vi "Measurement Logic.vi"() -> ()   [LabVIEW 2021, in "AC Dual Channel_Audio ADC.lvlib"]
uses:
  AC Dual Channel_Audio ADC.lvlib
  Measurement Configuration.ctl
  Measurement Results.ctl
  <vilib>/MeasurementLink/MeasurementLink Measurement Server/Measure Call Context/Measure Call Context.lvclass
  shared/controls/Sync Commands.ctl
  <vilib>/DAQmx/create/channels.llb/DAQmx Create Channel (AO-FuncGen).vi
  <vilib>/PDM Acquisition Toolkit/host/API/Public/Start/Start PCM Input Task.vi
  <vilib>/PDM Acquisition Toolkit/host/API/Public/Read/Read PCM Input Waveform.vi
  <vilib>/PDM Acquisition Toolkit/host/API/Public/Clear/Clear PCM Input Task.vi
  shared/controls/Audio ADC Controls.lvlib
  shared/Audio ADC Shared.lvlib
  <vilib>/PDM Acquisition Toolkit/host/API/PDM Acquisition Toolkit.lvlib
panel:
  out "measure call context out":refnum<class "Measure Call Context.lvclass">
  in  "measure call context in":refnum<class "Measure Call Context.lvclass">
  out "measurement results":T1
  in  "measurement configuration":T2={"Band start"=20.0, "Band stop"=20000.0, "Weighting Filter"=enum."Linear", "Full scale range"=2.825, "Left channel name"="", "Right channel name"="", "Left channel analog source resource name"="", "Right channel analog source resource name"="", "Frequency"=1000.0, "Amplitude"=-1.0, "Protocol capture resource name"="", "Data line"=0, "Left acquisition channel"=0, "Right acquisition channel"=0, "Sample rate"=44100.0, "Measurement Duration"=0.1, "Frame sync edge for Channel 0"=enum."Falling", "Channel count per frame"=2, "Channel length"=32, "Bit depth"=24, "Channel 0 offset"=1, "Endianness"=enum."MSB First", "Data Justification"=enum."Left Justified", "Frame length"=64, "Frame sync pulse width"=32, "Bit clock edge  sync"=enum."Falling"} {"Frame length" format="%#_6ps"}
  out "error out":errorcluster
  in  "error in":errorcluster
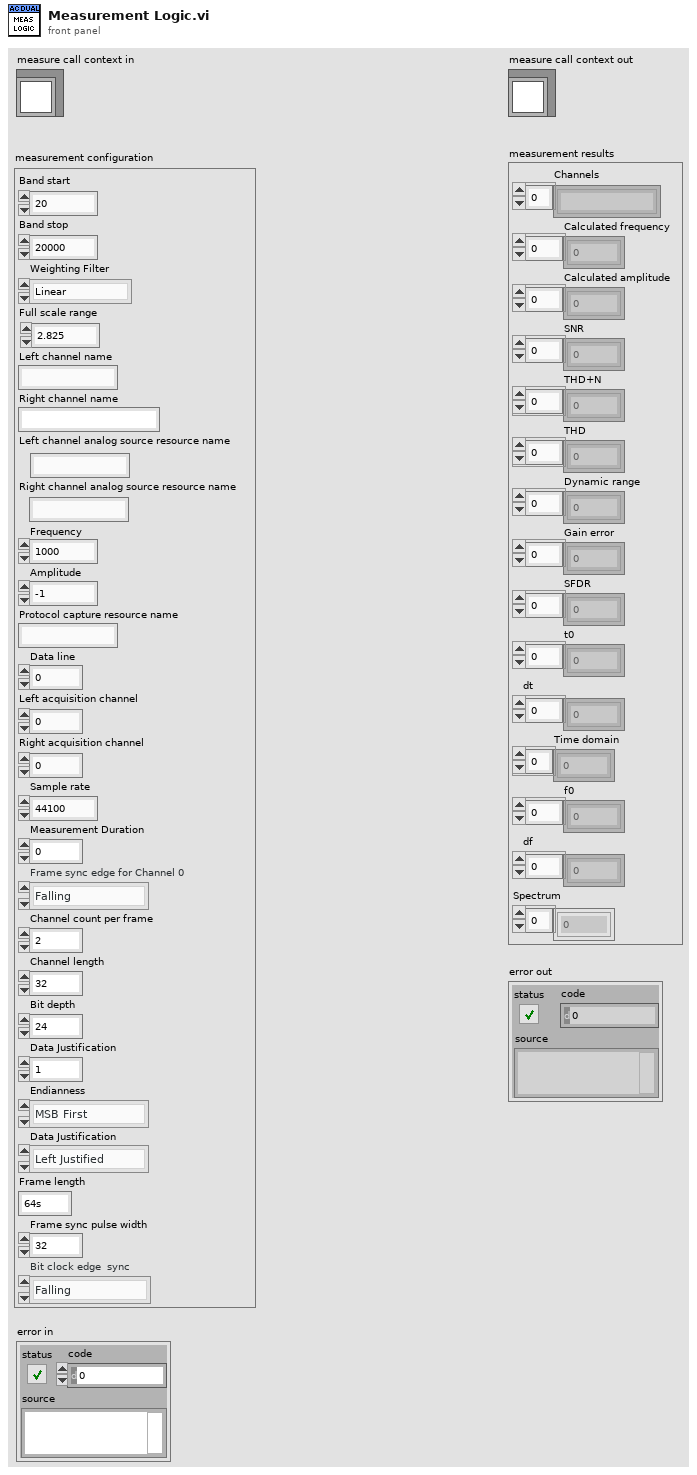
[diagram p1: front panel]
types:
  T1 = typedef "AC Dual Channel_Audio ADC.lvlib/Measurement Results.ctl" = cluster{"Channels":string[], "Calculated frequency":dbl[], "Calculated amplitude":dbl[], "SNR":dbl[], "THD+N":dbl[], "THD":dbl[], "Dynamic range":dbl[], "Gain error":dbl[], "SFDR":dbl[], "t0":dbl[], "dt":dbl[], "Time domain":dbl[], "f0":dbl[], "df":dbl[], "Spectrum":dbl[]}
  T2 = typedef "AC Dual Channel_Audio ADC.lvlib/Measurement Configuration.ctl" = cluster{"Band start":dbl, "Band stop":dbl, "Weighting Filter":enum32{"Linear", "A-weighting", "B-weighting", "C-weighting"}, "Full scale range":dbl, "Left channel name":string, "Right channel name":string, "Left channel analog source resource name":string, "Right channel analog source resource name":string, "Frequency":dbl, "Amplitude":dbl, "Protocol capture resource name":string, "Data line":i32, "Left acquisition channel":i32, "Right acquisition channel":i32, "Sample rate":dbl, "Measurement Duration":dbl, "Frame sync edge for Channel 0":enum32{"Rising", "Falling"}, "Channel count per frame":u32, "Channel length":u32, "Bit depth":u32, "Channel 0 offset":u32, "Endianness":enum32{"MSB First", "LSB First"}, "Data Justification":enum32{"Left Justified", "Right Justified"}, "Frame length":u32, "Frame sync pulse width":u32, "Bit clock edge  sync":enum32{"Rising", "Falling"}}
  T3 = typedef "audio adc controls.lvlib/Sync Commands.ctl" = enum16{"NoAction", "GenerationStarted", "AcquisitionCompleted", "GenerationErrored"}
  T4 = typedef "Audio ADC Controls.lvlib/Protocol Settings Dual Channel.ctl" = cluster{"Protocol capture resource name":string, "Data line":u16, "Channel":string, "Clock rate":u32, "Number of words":i32, "Sensitivity":dbl, "Frame sync edge for channel 0":enum32{"Rising", "Falling"}, "Channel count per frame":u8, "Channel length":u16, "Bit depth":u8, "Channel 0 offset":u16, "Endianness":enum32{"MSB First", "LSB First"}, "Data justification":enum32{"Left Justified", "Right Justified"}, "Frame length":u16, "Frame sync pulse width":u16, "Bit clock edge sync":enum32{"Rising", "Falling"}}
  T5 = typedef "PDM Acquisition Class Library.lvlib/PCM Input Task.lvclass/DVR PCM Input Task.ctl" = refnum<data-value>
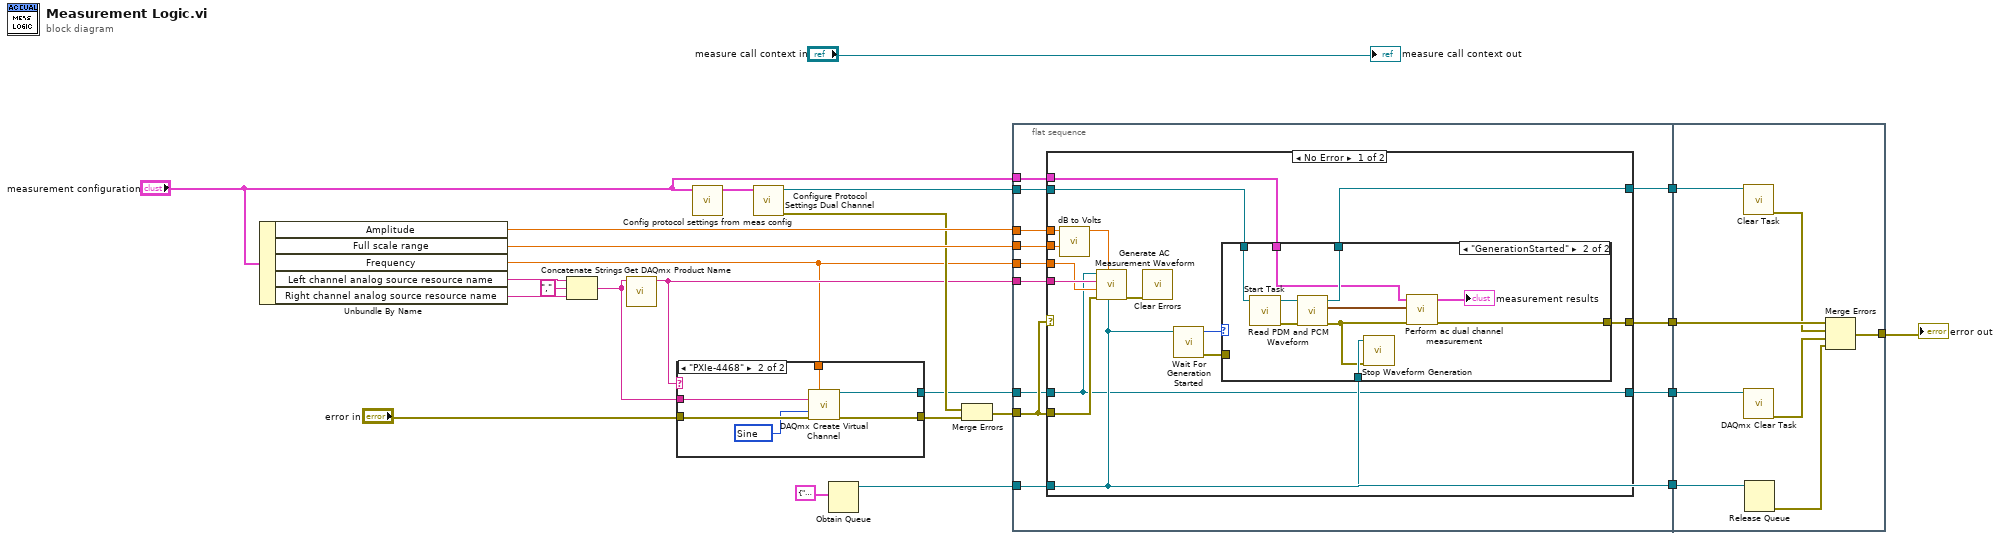
[diagram p0: block diagram]
diagram:
  n1 = Unbundle By Name("measurement configuration") -> ("Amplitude"=w19:dbl, "Full scale range"=w18:dbl, "Frequency"=w11:dbl, "Left channel analog source resource name"=w6:string, "Right channel analog source resource name"=w4:string)
  n2 = Concatenate Strings(w6, "," ("string"), w4) -> (w5:string)
  n3 = call "Get DAQmx Product Name.vi"("DAQmx resource name"=w5) -> ("DAQmx product type"=w12:string)  [unwired: 10 in]
  n4 = case shown="\"PXIe-4468\"" w12 {
    tunnel: w5 -> [_ w30]
    tunnel: "error in" -> [w25 w31]
    tunnel: [w25 w27] -> w16
    tunnel: w11 -> [_ w28]
    tunnel: [_ w26] -> w1
    frame Default {
    }
    frame "PXIe-4468" {
      w29 = 14751 items=["Sine"=14751, "Triangle"=14752, "Square"=14753, "Sawtooth"=14754] ("type")
      n5 = call-poly <vilib>:"DAQmx Create Virtual Channel.vi"("frequency"=w28, "physical channels"=w30, "type"=w29, "error in"=w31) -> ("task out"=w26:refnum<k21>, "error out"=w27:errorcluster)  [unwired: 10 in]
    }
  }
  n6 = call "Config protocol settings from meas config.vi"("measurement configuration"="measurement configuration") -> ("Protocol settings"=w8:T4)  [unwired: 10 in]
  n7 = call "Configure Protocol Settings Dual Channel.vi"("Protocol settings"=w8) -> ("error out"=w15:errorcluster, "PCM input task out"=w17:T5)  [unwired: 9 in]
  n8 = Obtain Queue(element data type=cluster{"Status":T3, "Error":errorcluster} {"Status"=enum."NoAction", "Error"={"status"=FALSE, "code"=0, "source"=""}}) -> (queue out=w13:refnum<queue>)  [unwired: 4 in, 2 out]
  n9 = Merge Errors(w15, w16) -> (w14:errorcluster)
  n10 = flat-sequence {
    tunnel: w19 -> [w43]
    tunnel: w18 -> [w42]
    tunnel: w13 -> [w40]
    tunnel: w14 -> [w34]
    tunnel: w17 -> [w41]
    tunnel: [w40] -> w23
    tunnel: [w38] -> w22
    tunnel: [w39] -> w21
    tunnel: w12 -> [w37]
    tunnel: w11 -> [w36]
    tunnel: "measurement configuration" -> [w35]
    tunnel: [w33] -> w2
    tunnel: w1 -> [w32]
    tunnel: w23 -> [w81]
    tunnel: w22 -> [w80]
    tunnel: w21 -> [w79]
    tunnel: [w75] -> w9
    tunnel: w2 -> [w74]
    frame #0 {
      n11 = case shown="No Error" w34 {
        selector: w34 -> [_ w72]
        tunnel: w43 -> [w58 _]
        tunnel: w42 -> [w57 _]
        tunnel: w34 -> [w54 _]
        tunnel: w41 -> [w53 w73]
        tunnel: w40 -> [w50 _]
        tunnel: [w49 w72] -> w39
        tunnel: [w48 w73] -> w38
        tunnel: w37 -> [w47 _]
        tunnel: w36 -> [w46 _]
        tunnel: w35 -> [w45 _]
        tunnel: [w44 w71] -> w33
        tunnel: w32 -> [w44 w71]
        frame No Error {
          n12 = call "dB to Volts.vi"("Full scale range"=w57, "Voltage(dB)"=w58) -> ("Voltage(volts)"=w56:dbl)  [unwired: 9 in]
          n13 = call "Generate AC Measurement Waveform.vi"("hardware commands sync queue"=w50, "Voltage(volts)"=w56, "error in"=w54, "Frequency"=w46, "DAQmx product name"=w47, "DSG task in"=w44) -> ("error out"=w55:errorcluster)  [unwired: 4 in, 1 out]
          n14 = call <vilib>:"Clear Errors.vi"("error in (no error)"=w55) -> ()  [unwired: 5 in, 2 out]
          n15 = call "Wait For Generation Started.vi"("hardware commands sync queue"=w50) -> ("error out"=w51:errorcluster, "Status"=w52:T3)  [unwired: 9 in]
          n16 = case shown="\"GenerationStarted\"" w52 {
            tunnel: w53 -> [w59 w68]
            tunnel: [w60 w65] -> w49
            tunnel: w51 -> [w60 _]
            tunnel: [w59 w67] -> w48
            tunnel: w50 -> [_ w66]
            tunnel: w45 -> [_ w63]
            frame Default {
            }
            frame "GenerationStarted" {
              n17 = call-poly <vilib>:"Start Task.vi"("PCM input task in"=w68) -> ("error out"=w70:errorcluster, "PCM input task out"=w69:T5)  [unwired: 9 in]
              n18 = call-poly <vilib>:"Read PDM and PCM Waveform.vi"("error in"=w70, "PCM input task In"=w69) -> ("error out"=w62:errorcluster, "PCM waveforms"=w64:waveform(dbl)[], "PCM input task out"=w67:T5)  [unwired: 4 in, 3 out]
              n19 = call "Stop Waveform Generation.vi"("error in (no error)"=w62, "Hw sync command Q"=w66) -> ()  [unwired: 10 in]
              n20 = call "Perform ac dual channel measurement.vi"("error in"=w62, "I2S waveforms"=w64, "measurement configuration"=w63) -> ("error out"=w65:errorcluster, "measurement results"=→"measurement results":T1)  [unwired: 7 in]
            }
          }
        }
        frame Error {
        }
      }
    }
    frame #1 {
      n21 = call-poly <vilib>:"Clear Task.vi"("PCM input task in"=w80) -> ("error out"=w78:errorcluster)  [unwired: 10 in]
      n22 = call <vilib>:"DAQmx Clear Task.vi"("task in"=w74) -> ("error out"=w77:errorcluster)  [unwired: 14 in]
      n23 = Release Queue(queue=w81) -> (error out=w76:errorcluster)  [unwired: 2 in, 2 out]
      n24 = Merge Errors(w79, w78, w77, w76) -> (w75:errorcluster)
    }
  }
  "error out" <- w9
  "measure call context out" <- "measure call context in"
